vi "airconditioner_better.vi"() -> ()   [LabVIEW 2026]
uses:
  <vilib>/numeric/Random Number (Range) I64.vi
  <vilib>/numeric/sub_Random U32.vi
panel:
  out "Numeric":i64
  out "Target Temperature 2":i64
  out "Enum":T1(ring)
  out "Current Room Temperature":i64(slide) scale=0.0..50.0
  in  "Confirm":bool
  in  "Target Temperature":i64(slide) scale=0.0..50.0
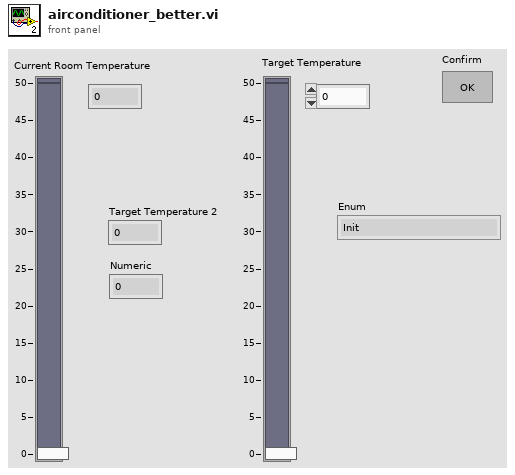
[diagram p1: front panel]
types:
  T1 = enum16{"Init", "Select Temperature", "Temperature Monitoring", "Cool", "Heat", "Exit"}
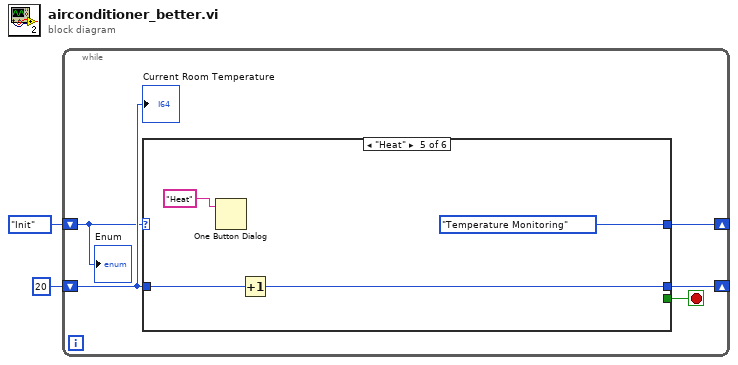
[diagram p0: block diagram]
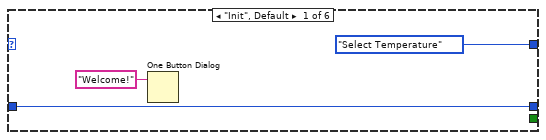
[diagram p2: hidden frame]
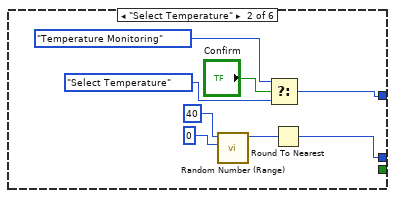
[diagram p3: hidden frame]
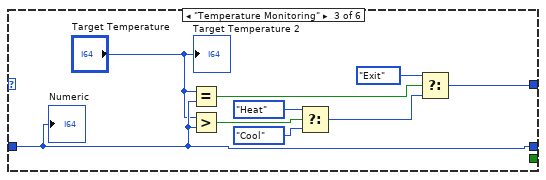
[diagram p4: hidden frame]
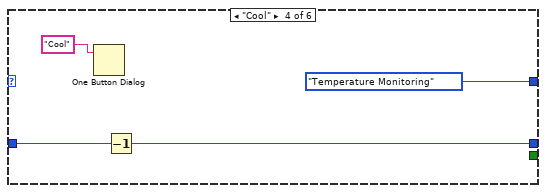
[diagram p5: hidden frame]
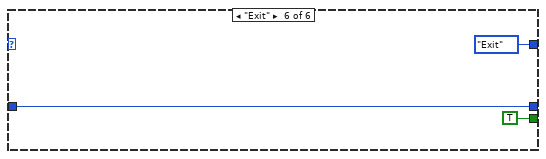
[diagram p6: hidden frame]
diagram:
  n1 = while {
    shift-right: [w7] -> _
    shift-left: T1."Init" -> [w3]
    shift-right: [w5] -> _
    shift-left: i64 20 -> [w4]
    stop <- w6 stop-if-true
    n2 = case shown="\"Heat\"" w3 {
      tunnel: [T1."Select Temperature" w16 w24 T1."Temperature Monitoring" T1."Temperature Monitoring" T1."Exit"] -> w7
      tunnel: [_ _ _ _ _ TRUE] -> w6
      tunnel: [w8 w14 w20 w29 w33 w36] -> w5
      tunnel: w4 -> [w8 _ w20 w30 w34 w36]
      frame "Init", Default {
        n3 = One Button Dialog(message="Welcome!") -> ()  [unwired: 1 in, 1 out]
      }
      frame "Select Temperature" {
        n4 = call-poly <vilib>:"Random Number (Range).vi"("lower bound (-100)"=i64 0, "upper bound (100)"=i64 40) -> ("number"=w13:i64)  [unwired: 9 in]
        n5 = Select(t=T1."Temperature Monitoring", s="Confirm", f=T1."Select Temperature") -> (s? t:f=w16:T1)
        n6 = Round To Nearest(number=w13) -> (nearest integer value=w14:i64)
      }
      frame "Temperature Monitoring" {
        n7 = Equal?(x="Target Temperature", y=w20) -> (x = y?=w21:bool)
        n8 = Greater?(x="Target Temperature", y=w20) -> (0:w26:bool)
        n9 = Select(t=T1."Heat", s=w26, f=T1."Cool") -> (s? t:f=w23:T1)
        n10 = Select(t=T1."Exit", s=w21, f=w23) -> (s? t:f=w24:T1)
        "Target Temperature 2" <- "Target Temperature"
        "Numeric" <- w20
      }
      frame "Cool" {
        n11 = One Button Dialog(message="Cool") -> ()  [unwired: 1 in, 1 out]
        n12 = Decrement(x=w30) -> (x-1=w29:i64)
      }
      frame "Heat" {
        n13 = One Button Dialog(message="Heat") -> ()  [unwired: 1 in, 1 out]
        n14 = Increment(x=w34) -> (x+1=w33:i64)
      }
      frame "Exit" {
      }
    }
    "Current Room Temperature" <- w4
    "Enum" <- w3
  }
